vi "CLSUIP_CreateNewAccessor.vi"(4 "Make available through Property Nodes":bool, 5 "VI Type":enum32{"Dynamic", "Static"}(ring)=enum."Static", 6 "Include error terminals":bool, 7 "Virtual Folder Name":string, 8 "error in (no error)":errorcluster, 9 "Access UI":T1, 10 "PDC Item Refnum":refnum<vi>, 11 "LVClassLibrary Ref":refnum<vi>) -> (0 "error out":errorcluster, 1 "Write VI":refnum<vi>, 2 "Read VI":refnum<vi>)   [LabVIEW 2021, in "MemberVICreation.lvlib"]
uses:
  <resource>/Framework/Providers/LVClassLibrary/NewAccessors/MemberVICreation.lvlib
  <resource>/Framework/Providers/LVClassLibrary/NewAccessors/CLSUIP_Access.ctl
  <resource>/Framework/Providers/LVClassLibrary/NewAccessors/BaseAccessorScripter/BaseAccessorScripter.lvclass
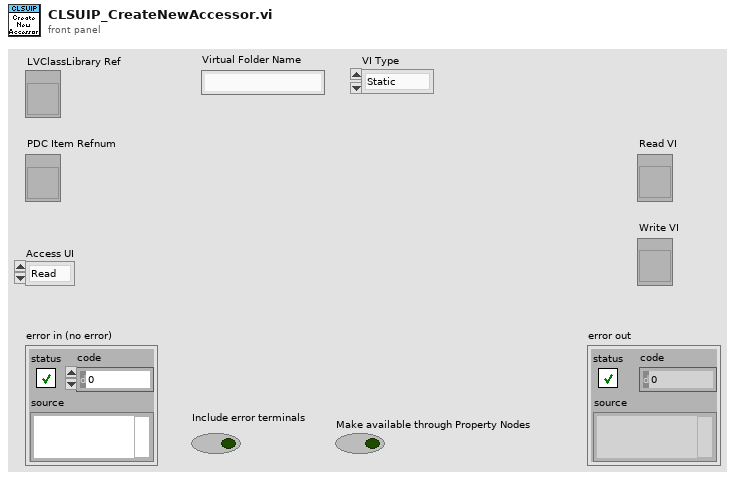
[diagram p1: front panel]
types:
  T1 = typedef "MemberVICreation.lvlib/CLSUIP_Access.ctl" = enum16{"Read", "Write", "R/W"}
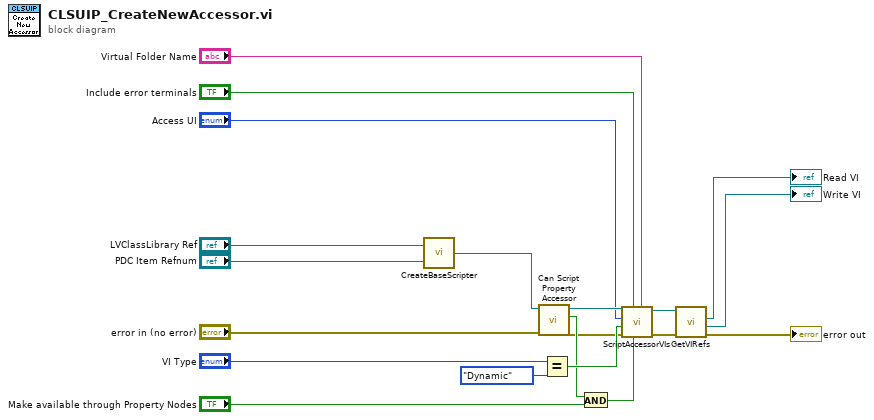
[diagram p0: block diagram]
diagram:
  n1 = call <resource>:"CreateBaseScripter.vi"("Ctl Refnum"="PDC Item Refnum", "LVClassLibrary Ref"="LVClassLibrary Ref") -> ("Scripter Out"=w6:refnum<class "BaseAccessorScripter.lvclass">)
  n2 = call-dynamic "Can Script Property Accessor.vi"("error in (no error)"="error in (no error)", "BaseAccessorScripter in"=w6) -> ("error out"=w14:errorcluster, "Can Script Property Accessor"=w16:bool, "BaseAccessorScripter out"=w15:refnum<class "BaseAccessorScripter.lvclass">)  [unwired: 7 in]
  n3 = Equal?(x="VI Type", y=enum32{"Dynamic", "Static"}."Dynamic") -> (x = y?=w19:bool)
  n4 = And(x=w16, y="Make available through Property Nodes") -> (x .and. y?=w13:bool)
  n5 = call-dynamic "ScriptAccessorVIs.vi"("Virtual Folder Name"="Virtual Folder Name", "Create as Properties"=w13, "Include error terminals"="Include error terminals", "error in (no error)"=w14, "Make Class Terminals Dynamic"=w19, "Access"="Access UI", "BaseAccessorScripter in"=w15) -> ("error out"=w17:errorcluster, "BaseAccessorScripter out"=w18:refnum<class "BaseAccessorScripter.lvclass">)  [unwired: 3 in]
  n6 = call-dynamic "GetVIRefs.vi"("error in (no error)"=w17, "BaseAccessorScripter in"=w18) -> ("error out"=→"error out":errorcluster, "Write VI"=→"Write VI":refnum<vi>, "Read VI"=→"Read VI":refnum<vi>)  [unwired: 6 in, 1 out]
